vi "AM mod(SubVI).vi"(1 "signal in":waveform(dbl), 3 "carrier frequency":dbl(knob)=10.0 scale=0.0..500000.0) -> (0 "modulated signal (time-domain)":waveform(dbl)(graph))   [LabVIEW 2010]
uses:
  <vilib>/measure/NI_MABase.lvlib
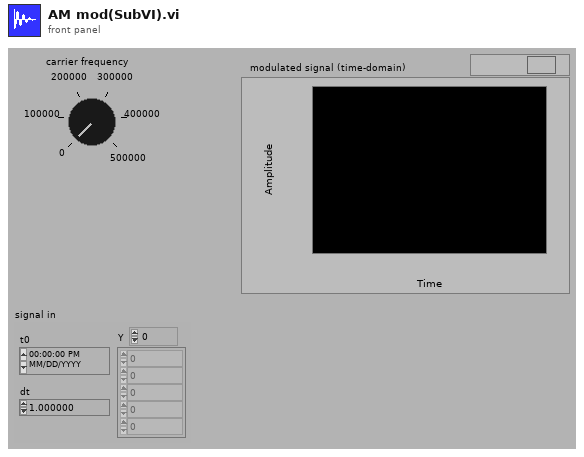
[diagram p1: front panel]
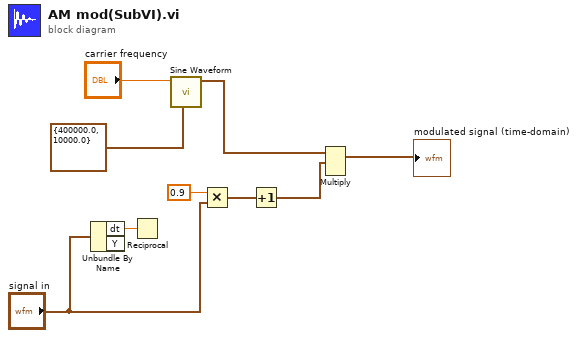
[diagram p0: block diagram]
diagram:
  n1 = Unbundle By Name("signal in") -> ("dt"=w1:dbl)  [unwired: 1 out]
  n2 = Reciprocal(x=w1) -> ()  [unwired: 1 out]
  n3 = call <vilib>:"Sine Waveform.vi"("sampling info"=cluster{"Fs":dbl, "#s":dbl} {"Fs"=400000.0, "#s"=10000.0}, "frequency"="carrier frequency") -> ("signal out"=w5:waveform(dbl))  [unwired: 8 in, 1 out]
  n4 = Multiply(x=0.9, y="signal in") -> (x*y=w8:waveform(dbl))
  n5 = Increment(x=w8) -> (x+1=w6:waveform(dbl))
  n6 = Multiply(1:w6, 2:w5) -> (0:→"modulated signal (time-domain)":waveform(dbl))  [unwired: 1 in, 1 out]
